vi "NGTS_Find_Number_Of_PID_Loops.vi"(8 "error in":errorcluster, 10 "Search String":string="PID_", 11 "Tags":string[](array[string])=["MFC390LSP_CO", "MFC390HSP_CO", "MFC660LSP_H2", "MFC660HSP_H2", "HTR660SP", "HTR661SP", "HTR662SP", "MFC760LSP_N2", "MFC760HSP_N2", "MFC160LSP_O2", "MFC160HSP_O2", "MFC380LSP_CO2", "MFC380HSP_CO2", "MFC260LSP_CH4", "MFC260HSP_CH4", "CV760_N2", "CV460", "CV462", "CV461", "CV661", "CV160L_O2", "CV160H_O2", "CV760L_N2", "CV760H_N2", "CV380L_CO2", "CV380H_CO2", "CV260L_CH4", "CV260H_CH4", "CV390L_CO", "CV390H_CO", "CV660L_H2", "HTR660E", "HTR660RST", "HTR661E", "HTR661RST", "HTR662E", "HTR662RST", "PMP460", "PMP461", "DATE", "TIME", "ONLOAD_TIME", "H2UTIL", "O2UTIL", "CELL", "VT_AVG", "VT_MIN", "VT_MAX", "SD1_BP", "SD1_A", "SD1_B", "SD1_C", "SD1_D", "SDOUT", "AN_DR_SAT", "AN_SAT_MIN_FL", "AN_SAT_TOT_FL", "PCV662SP", "PMP440_SELECT", "PMP441_SELECT", "MFC760SP_N2", "MFC760LSP_N2_MAX", "CV760L", "CV760H", "MFC760_N2", "MFC760LSP_N2", "MFC760HSP_N2", "PID_001_SP", "PID_001_FB", "PID_001_OUT", "PID_001_UPD", "PID_001_OUTH", "PID_001_OUTL", "PID_001_AM", "PID_001_ERR", "PID_001_P", "PID_001_I", "PID_001_D", "PID_001_BUMP", "PID_001_SPMAX", "PID_001_MIN", "PID_002_SP", "PID_002_FB", "PID_002_OUT", "PID_002_UPD"]) -> (0 "error out":errorcluster, 2 "PID Loop Names":string[](array[string]), 3 "PID Tags":string[](array[string]), 5 "PID Loops":i32)   [LabVIEW 2010]
doc: "Searchs a list of Tag names and returns a filtered list of PID related Tags, the number of total PID loops found and an array of the PID loop numbers.\n\nThe search string defaults to: PID_[0-9]+_\n\nThis searchs for all tags with a number between the underscores. The number is extracted and added to an array, which is then filtered to remove duplicate numbers. In this way, the PID loop numbers do not have to be contiguous, ie you could have loop numbers 1, 4 and 7.\n\nThis may be easily upgraded to identify PID loops based on a Loop Name rather than a number. Currently eachset of PID parameter Tags is identified by a loop number, beginning at 1.\n\n2008_01_09 Mike Ashe\nmichael.ashe@imaginatics.net\nCell: 860-961-0876"
uses:
  <userlib>/_OpenG.lib/array/array.llb/Remove Duplicates from 1D Array (String)__ogtk.vi
panel:
  # "Find PID Loops from Tag List by TekTHINK"
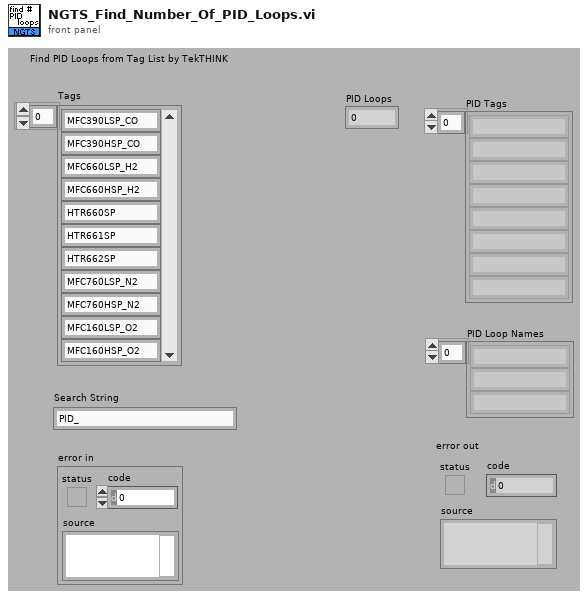
[diagram p1: front panel]
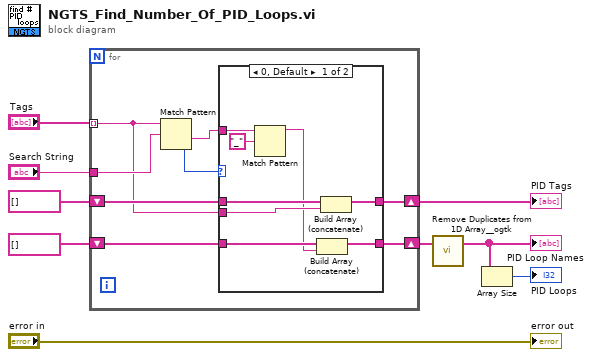
[diagram p0: block diagram]
diagram:
  n1 = for {
    tunnel: "Search String" -> [w15]
    tunnel: "Tags" -> [w13] mode=indexing
    shift-right: [w14] -> w8
    shift-left: string[] [] -> [w16]
    shift-right: [w12] -> w3
    shift-left: string[] [] -> [w11]
    n2 = Match Pattern(string=w13, regular expression=w15) -> (after substring=w10:string, offset past match=w17:i32)  [unwired: 1 in, 2 out]
    n3 = case shown="0, Default" w17 {
      tunnel: w16 -> [w25 w27]
      tunnel: w13 -> [w24 _]
      tunnel: [w23 w27] -> w14
      tunnel: w10 -> [w20 _]
      tunnel: w11 -> [w21 w26]
      tunnel: [w22 w26] -> w12
      frame 0, Default {
        n4 = Match Pattern(string=w20, regular expression="_") -> (before substring=w18:string)  [unwired: 1 in, 3 out]
        n5 = Build Array (concatenate)(w21, w18) -> (w22:string[])
        n6 = Build Array (concatenate)(w25, w24) -> (w23:string[])
      }
      frame -1 {
      }
    }
  }
  "PID Tags" <- w8
  n7 = call-poly <userlib>:"Remove Duplicates from 1D Array__ogtk.vi"("Input Array"=w3) -> ("Output Array"=w2:string[])  [unwired: 1 out]
  "PID Loop Names" <- w2
  n8 = Array Size(array=w2) -> (size(s)=→"PID Loops":i32)
  "error out" <- "error in"
